vi "IsInRange.vi"(8 "标称量":dbl, 11 "输入量":dbl) -> (0 "范围内？":bool)   [LabVIEW 2009]
doc: "判断输入量是否在标称量+/-10%范围内"
panel:
  out "error out":errorcluster
  in  "error in (no error)":errorcluster
  # "判断输入量是否在标称量+/-10%范围内"
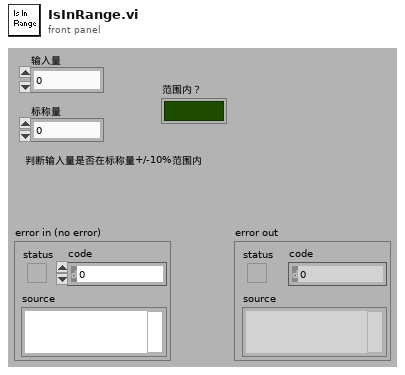
[diagram p1: front panel]
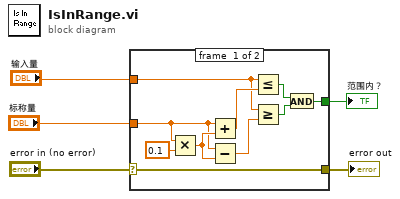
[diagram p0: block diagram]
diagram:
  n1 = case shown="Error" "error in (no error)" {
    selector: "error in (no error)" -> [w9 w16]
    tunnel: [w9 w16] -> w4
    tunnel: "输入量" -> [w8 _]
    tunnel: "标称量" -> [w7 _]
    tunnel: [w6 _] -> w1
    frame #0 {
      n2 = Multiply(x=w7, y=0.1) -> (x*y=w14:dbl)
      n3 = Add(x=w7, y=w14) -> (x+y=w13:dbl)
      n4 = Subtract(x=w7, y=w14) -> (x-y=w12:dbl)
      n5 = Less Or Equal?(x=w8, y=w13) -> (x <= y?=w11:bool)
      n6 = Greater Or Equal?(x=w8, y=w12) -> (x >= y?=w10:bool)
      n7 = And(x=w11, y=w10) -> (x .and. y?=w6:bool)
    }
    frame #1 {
      # "错误时不做任何工作"
    }
  }
  "error out" <- w4
  "范围内？" <- w1
